vi "Update Focus Chart.vi"(6 "Refnums":T1, 8 "error in (no error)":errorcluster, 9 "Current Z":dbl, 10 "Target Data":T4, 11 "Focus Curve":T3) -> (0 "error out":errorcluster, 3 "Focus Plot":cluster{"Z (um)":dbl[], "Score":sgl[]}[](array[cluster]))   [LabVIEW 2014]
uses:
  AutoFocus Refnums.ctl
  support/Instrument Status.ctl
  ZScan.ctl
  <vilib>/Analysis/Matrix/Datatypes/RealMatrix.ctl
  Target Refnums.ctl
  <vilib>/Analysis/Matrix/NI_Matrix.lvlib
panel:
  # "LICENSED MATERIALS – PROPERTY OF IBM\nCopyright IBM Corp. 2016,\nALL RIGHTS RESERVED"
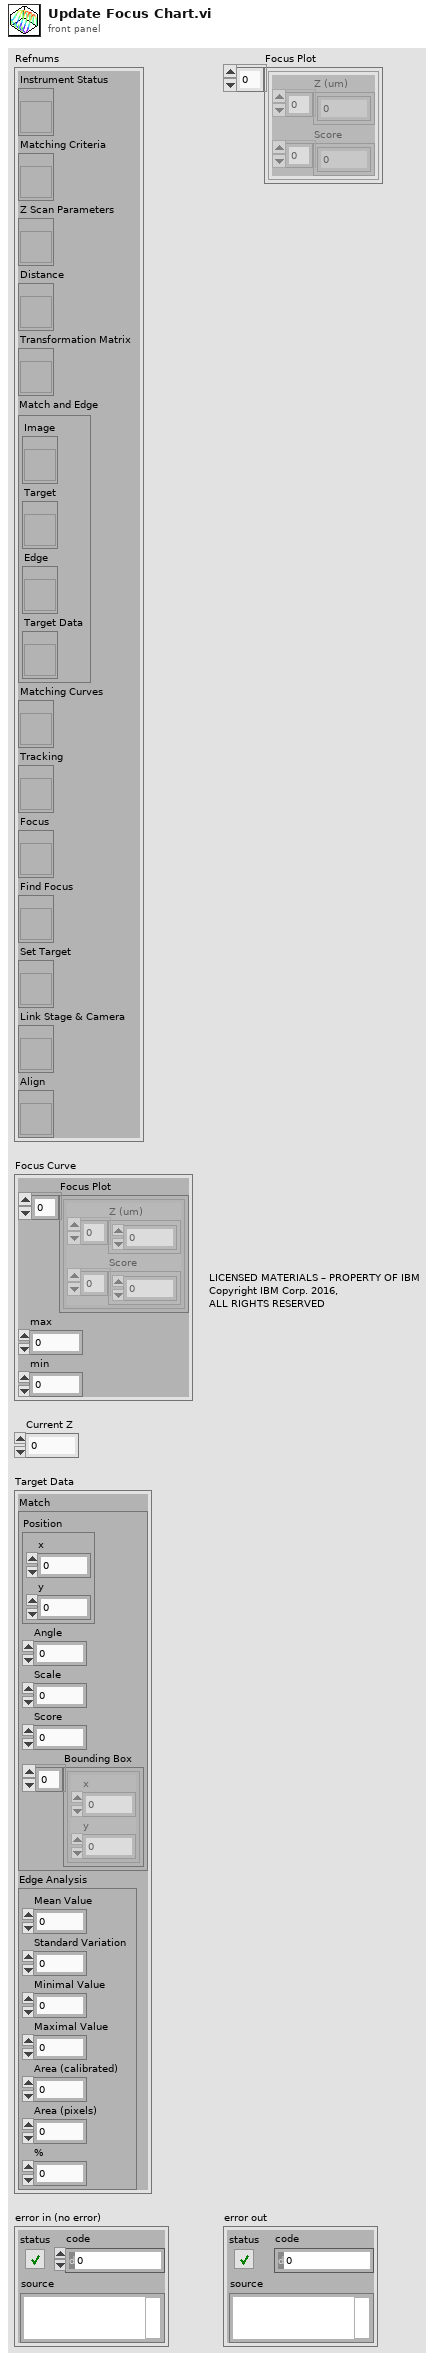
[diagram p1: front panel]
types:
  T1 = typedef "AutoFocus Refnums.ctl" = cluster{"Instrument Status":refnum<vi>, "Matching Criteria":refnum<vi>, "Z Scan Parameters":refnum<vi>, "Distance":refnum<vi>, "Transformation Matrix":refnum<vi>, "Match and Edge":T2, "Matching Curves":refnum<vi>, "Tracking":refnum<vi>, "Focus":refnum<vi>, "Find Focus":refnum<vi>, "Set Target":refnum<vi>, "Link Stage & Camera":refnum<vi>, "Align":refnum<vi>}
  T2 = typedef "Target Refnums.ctl" = cluster{"Image":refnum<vi>, "Target":refnum<vi>, "Edge":refnum<vi>, "Target Data":refnum<vi>}
  T3 = cluster{"Focus Plot":cluster{"Z (um)":dbl[], "Score":sgl[]}[], "max":sgl, "min":sgl}
  T4 = cluster{"Match":cluster{"Position":cluster{"x":sgl, "y":sgl}, "Angle":sgl, "Scale":sgl, "Score":sgl, "Bounding Box":cluster{"x":sgl, "y":sgl}[]}, "Edge Analysis":cluster{"Mean Value":sgl, "Standard Variation":sgl, "Minimal Value":sgl, "Maximal Value":sgl, "Area (calibrated)":sgl, "Area (pixels)":i32, "%":sgl}}
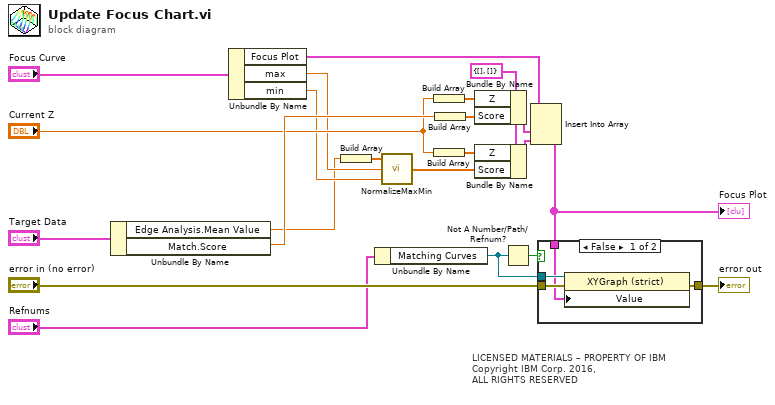
[diagram p0: block diagram]
diagram:
  w14 = cluster{"Z":dbl[], "Score":sgl[]} {"Z"=[], "Score"=[]} ("Function Out")
  # "LICENSED MATERIALS – PROPERTY OF IBM\nCopyright IBM Corp. 2016,\nALL RIGHTS RESERVED"
  n1 = Unbundle By Name("Target Data") -> ("Edge Analysis.Mean Value"=w1:sgl, "Match.Score"=w22:sgl)
  n2 = Unbundle By Name("Focus Curve") -> ("Focus Plot"=w8:cluster{"Z (um)":dbl[], "Score":sgl[]}[], "max"=w15:sgl, "min"=w16:sgl)
  n3 = Build Array(w1) -> (w2:sgl[])
  n4 = Unbundle By Name("Refnums") -> ("Matching Curves"=w3:refnum<vi>)
  n5 = call "NormalizeMaxMin.vi"("Min"=w16, "Max"=w15, "Score"=w2) -> ("Array"=w17:sgl[])
  n6 = Build Array("Current Z") -> (w10:dbl[])
  n7 = Build Array("Current Z") -> (w12:dbl[])
  n8 = Build Array(w22) -> (w11:sgl[])
  n9 = Bundle By Name(cluster=w14, "Z"=w10, "Score"=w11) -> (w9:cluster{"Z":dbl[], "Score":sgl[]})
  n10 = Bundle By Name(cluster=w14, "Z"=w12, "Score"=w17) -> (w13:cluster{"Z":dbl[], "Score":sgl[]})
  n11 = Not A Number/Path/Refnum?(number/path/refnum=w3) -> (NaN/Path/Refnum?=w4:bool)
  n12 = Insert Into Array(array=w8, new element #1=w9, new element #2=w13) -> (w18:cluster{"Z (um)":dbl[], "Score":sgl[]}[])  [unwired: 1 in]
  "Focus Plot" <- w18
  n13 = case shown="False" w4 {
    tunnel: "error in (no error)" -> [w26 w27]
    tunnel: [w25 w27] -> w19
    tunnel: w3 -> [w24 _]
    tunnel: w18 -> [w23 _]
    frame False {
      n14 = property class="XYGraph (strict)"(reference=w24, error in=w26, "Value"=w23) -> (error out=w25:errorcluster)  [unwired: 1 out]
    }
    frame True {
    }
  }
  "error out" <- w19
